vi "dfd_Update Wfm Time Stamp.vi"(7 "init? (F)":bool, 9 "signal in":waveform(dbl)={"t0"=timestamp(0 s since 1904-01-01), "dt"=0.0, "Y"=[]}, 11 "t0":timestamp) -> (1 "signal out":waveform(dbl), 3 "tf":timestamp)   [LabVIEW 2017, in "NI_DigFilterLicensed.lvlib"]
uses:
  <vilib>/addons/Digital Filter Design/NI_DigFilterLicensed.lvlib
  <vilib>/Waveform/WDTOps.llb/WDT Get Final Time Value DBL.vi
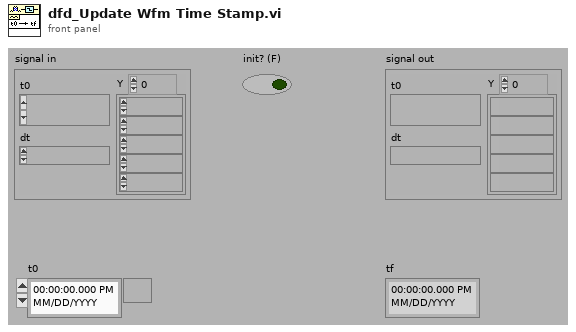
[diagram p1: front panel]
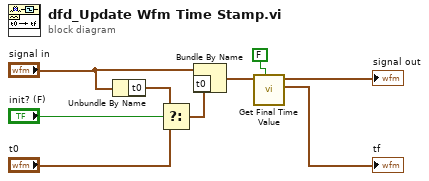
[diagram p0: block diagram]
diagram:
  n1 = Unbundle By Name("signal in") -> ("t0"=w4:timestamp)
  n2 = Select(t=w4, s="init? (F)", f="t0") -> (s? t:f=w3:timestamp)
  n3 = Bundle By Name(cluster="signal in", "t0"=w3) -> (w2:waveform(dbl))
  n4 = call-poly <vilib>:"Get Final Time Value.vi"("open interval? (T)"=FALSE, "waveform in"=w2) -> ("tf"=→"tf":timestamp, "waveform out"=→"signal out":waveform(dbl))  [unwired: 1 in, 7 out]
